vi "Generate Setter VI.vi"(7 "Highlight changes?":bool=TRUE, 8 "error in (no error)":errorcluster, 9 "class path":path, 10 "Attribute Name":string) -> (0 "error out":errorcluster)   [LabVIEW 2020, in "Method Generation.lvlib" / "Setter Generator.lvclass"]
uses:
  Setter Generator.lvclass
  Setter Generator.lvclass/Setter Generator.ctl
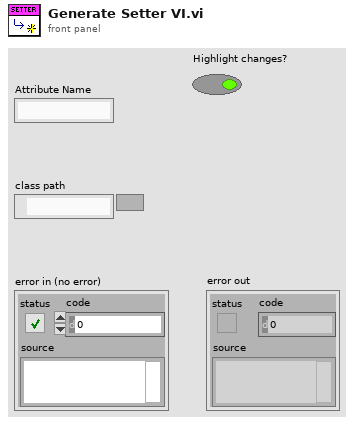
[diagram p1: front panel]
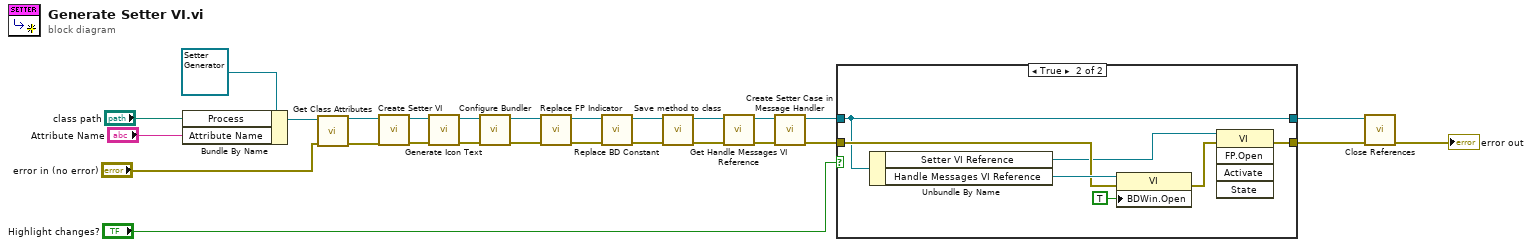
[diagram p0: block diagram]
diagram:
  n1 = Bundle By Name(cluster=refnum<class "Setter Generator.lvclass"> refnum ("New Getter Dialog In"), "Process"="class path", "Attribute Name"="Attribute Name") -> (w19:refnum<class "Setter Generator.lvclass">)
  n2 = call "Get Class Attributes.vi"("error in (no error)"="error in (no error)", "Setter Generator In"=w19) -> ("error out"=w23:errorcluster, "Setter Generator Out"=w22:refnum<class "Setter Generator.lvclass">)  [unwired: 8 in]
  n3 = call "Create Setter VI.vi"("error in (no error)"=w23, "Setter Generator In"=w22) -> ("error out"=w25:errorcluster, "Setter Generator Out"=w2:refnum<class "Setter Generator.lvclass">)  [unwired: 8 in]
  n4 = call "Generate Icon Text.vi"("error in (no error)"=w25, "Setter Generator In"=w2) -> ("error out"=w3:errorcluster, "Setter Generator Out"=w1:refnum<class "Setter Generator.lvclass">)  [unwired: 8 in]
  n5 = call "Configure Bundler.vi"("error in (no error)"=w3, "Setter Generator In"=w1) -> ("error out"=w17:errorcluster, "Setter Generator Out"=w26:refnum<class "Setter Generator.lvclass">)  [unwired: 8 in]
  n6 = call "Replace FP Indicator.vi"("error in (no error)"=w17, "Setter Generator In"=w26) -> ("error out"=w16:errorcluster, "Setter Generator Out"=w27:refnum<class "Setter Generator.lvclass">)  [unwired: 8 in]
  n7 = call "Replace BD Constant.vi"("error in (no error)"=w16, "Setter Generator In"=w27) -> ("error out"=w14:errorcluster, "Setter Generator Out"=w13:refnum<class "Setter Generator.lvclass">)  [unwired: 8 in]
  n8 = call "Save method to class.vi"("error in (no error)"=w14, "Setter Generator In"=w13) -> ("error out"=w10:errorcluster, "Setter Generator Out"=w11:refnum<class "Setter Generator.lvclass">)  [unwired: 8 in]
  n9 = call "Get Handle Messages VI Reference.vi"("error in (no error)"=w10, "Setter Generator In"=w11) -> ("error out"=w12:errorcluster, "Setter Generator Out"=w9:refnum<class "Setter Generator.lvclass">)  [unwired: 8 in]
  n10 = call "Create Setter Case in Message Handler.vi"("error in (no error)"=w12, "Setter Generator In"=w9) -> ("error out"=w8:errorcluster, "Setter Generator Out"=w5:refnum<class "Setter Generator.lvclass">)  [unwired: 8 in]
  n11 = case shown="True" "Highlight changes?" {
    tunnel: w5 -> [w28 w30]
    tunnel: w8 -> [w29 w34]
    tunnel: [w29 w32] -> w7
    tunnel: [w28 w30] -> w4
    frame False {
    }
    frame True {
      n12 = Unbundle By Name(w30) -> ("Setter VI Reference"=w31:refnum<vi>, "Handle Messages VI Reference"=w36:refnum<vi>)
      n13 = property class="VI"(reference=w36, error in=w34, "BDWin.Open"=TRUE ("Block Diagram Window:Open")) -> (error out=w33:errorcluster)  [unwired: 1 out]
      n14 = invoke class="VI" method="FP.Open"(reference=w31, error in=w33) -> (error out=w32:errorcluster)  [unwired: 3 in, 4 out]
    }
  }
  n15 = call "Close References.vi"("error in (no error)"=w7, "Setter Generator In"=w4) -> ("error out"=→"error out":errorcluster)  [unwired: 9 in]
